vi "SetOccurrence.vi"(2 "occurrence":refnum<k4>) -> ()   [LabVIEW 2019, in "_ChannelSupport.lvlib"]
uses:
  _ChannelSupport.lvlib
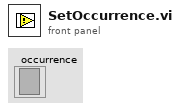
[diagram p1: front panel]
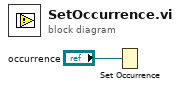
[diagram p0: block diagram]
diagram:
  n1 = Set Occurrence("occurrence") -> ()
